vi "CAN_initialize_all.vi"() -> (3 "Array of Canopen Sessions":refnum<class "sbCANopenBaseClass.lvclass">[](array[class]), 6 "Array of Error out's":errorcluster[](array[cluster]))   [LabVIEW 2024]
uses:
  <vilib>/addons/Maxon Motor/EPOS2 CANopen/CANopen/sbCANopenBaseClass.lvclass
  <vilib>/addons/Maxon Motor/EPOS2 CANopen/EPOS2 Support Files/Typedefs/EPOS2 Config Data Input Current.ctl
  <vilib>/addons/Maxon Motor/EPOS2 CANopen/EPOS2 Support Files/Typedefs/EPOS2 Velocity Units.ctl
  <vilib>/addons/Maxon Motor/EPOS2 CANopen/EPOS2 Support Files/Typedefs/EPOS2 Control Word PVM.ctl
  <vilib>/addons/Maxon Motor/EPOS2 CANopen/EPOS2 Support Files/Polymorphic SubVIs/Config/EPOS2 Current Mode Configure.vi
  <vilib>/addons/Maxon Motor/EPOS2 CANopen/EPOS2 Support Files/Polymorphic SubVIs/Write PDO/EPOS2 Current Mode Write.vi
  <vilib>/addons/Maxon Motor/EPOS2 CANopen/EPOS2 Library.lvlib
  <vilib>/addons/Maxon Motor/EPOS2 CANopen/CANopen/CANopen IndCom Interface/sdCANopenIndCom.lvclass
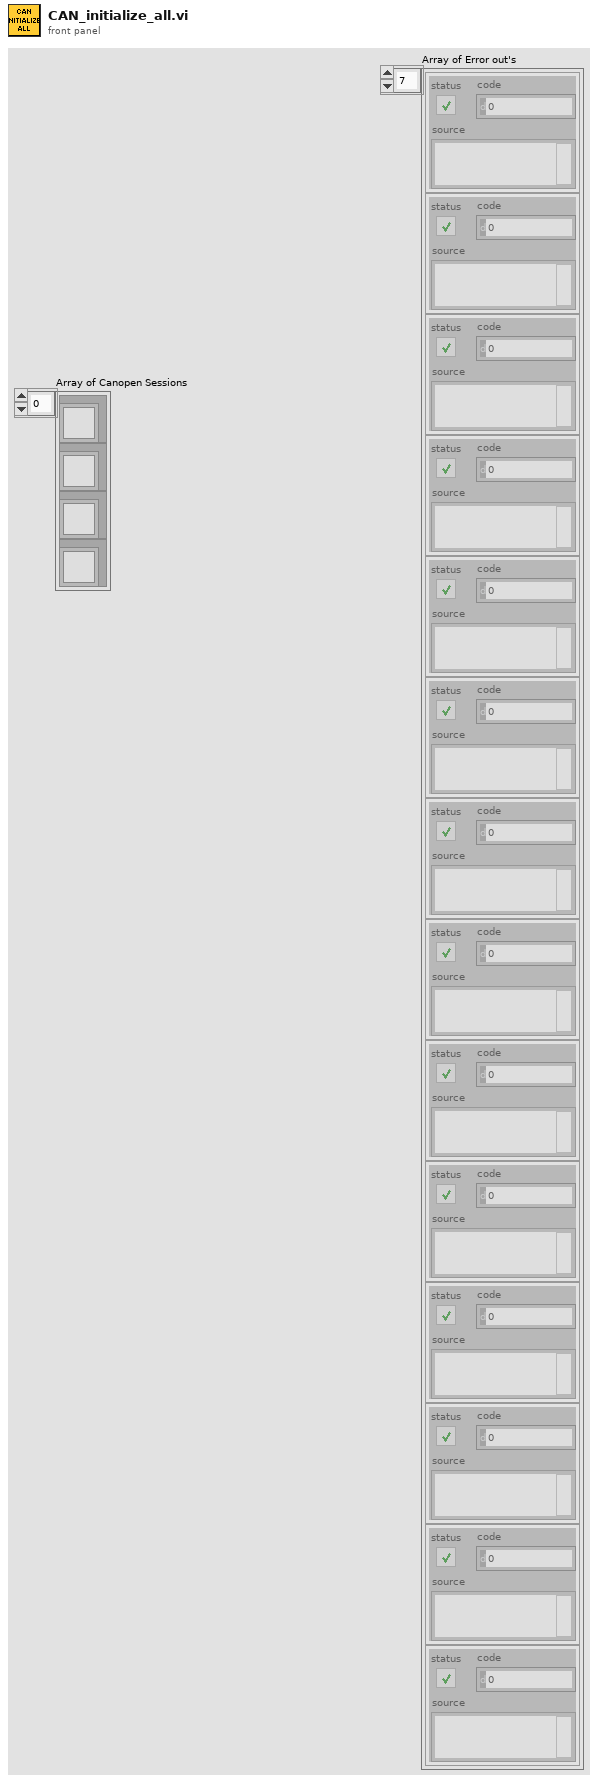
[diagram p1: front panel]
types:
  T1 = typedef "EPOS2 Library.lvlib/EPOS2 Control Word PVM.ctl" = cluster{"Switch On":bool, "Enable Voltage":bool, "Quick Stop":bool, "Enable Operation":bool, "Reserved 0":bool, "Reserved 1":bool, "Reserved 2":bool, "Fault Reset":bool, "Halt":bool}
  T2 = typedef "EPOS2 Library.lvlib/EPOS2 Config Data Input Current.ctl" = cluster{"Velocity Units":T3, "Max Velocity":i32}
  T3 = typedef "EPOS2 Library.lvlib/EPOS2 Velocity Units.ctl" = i8
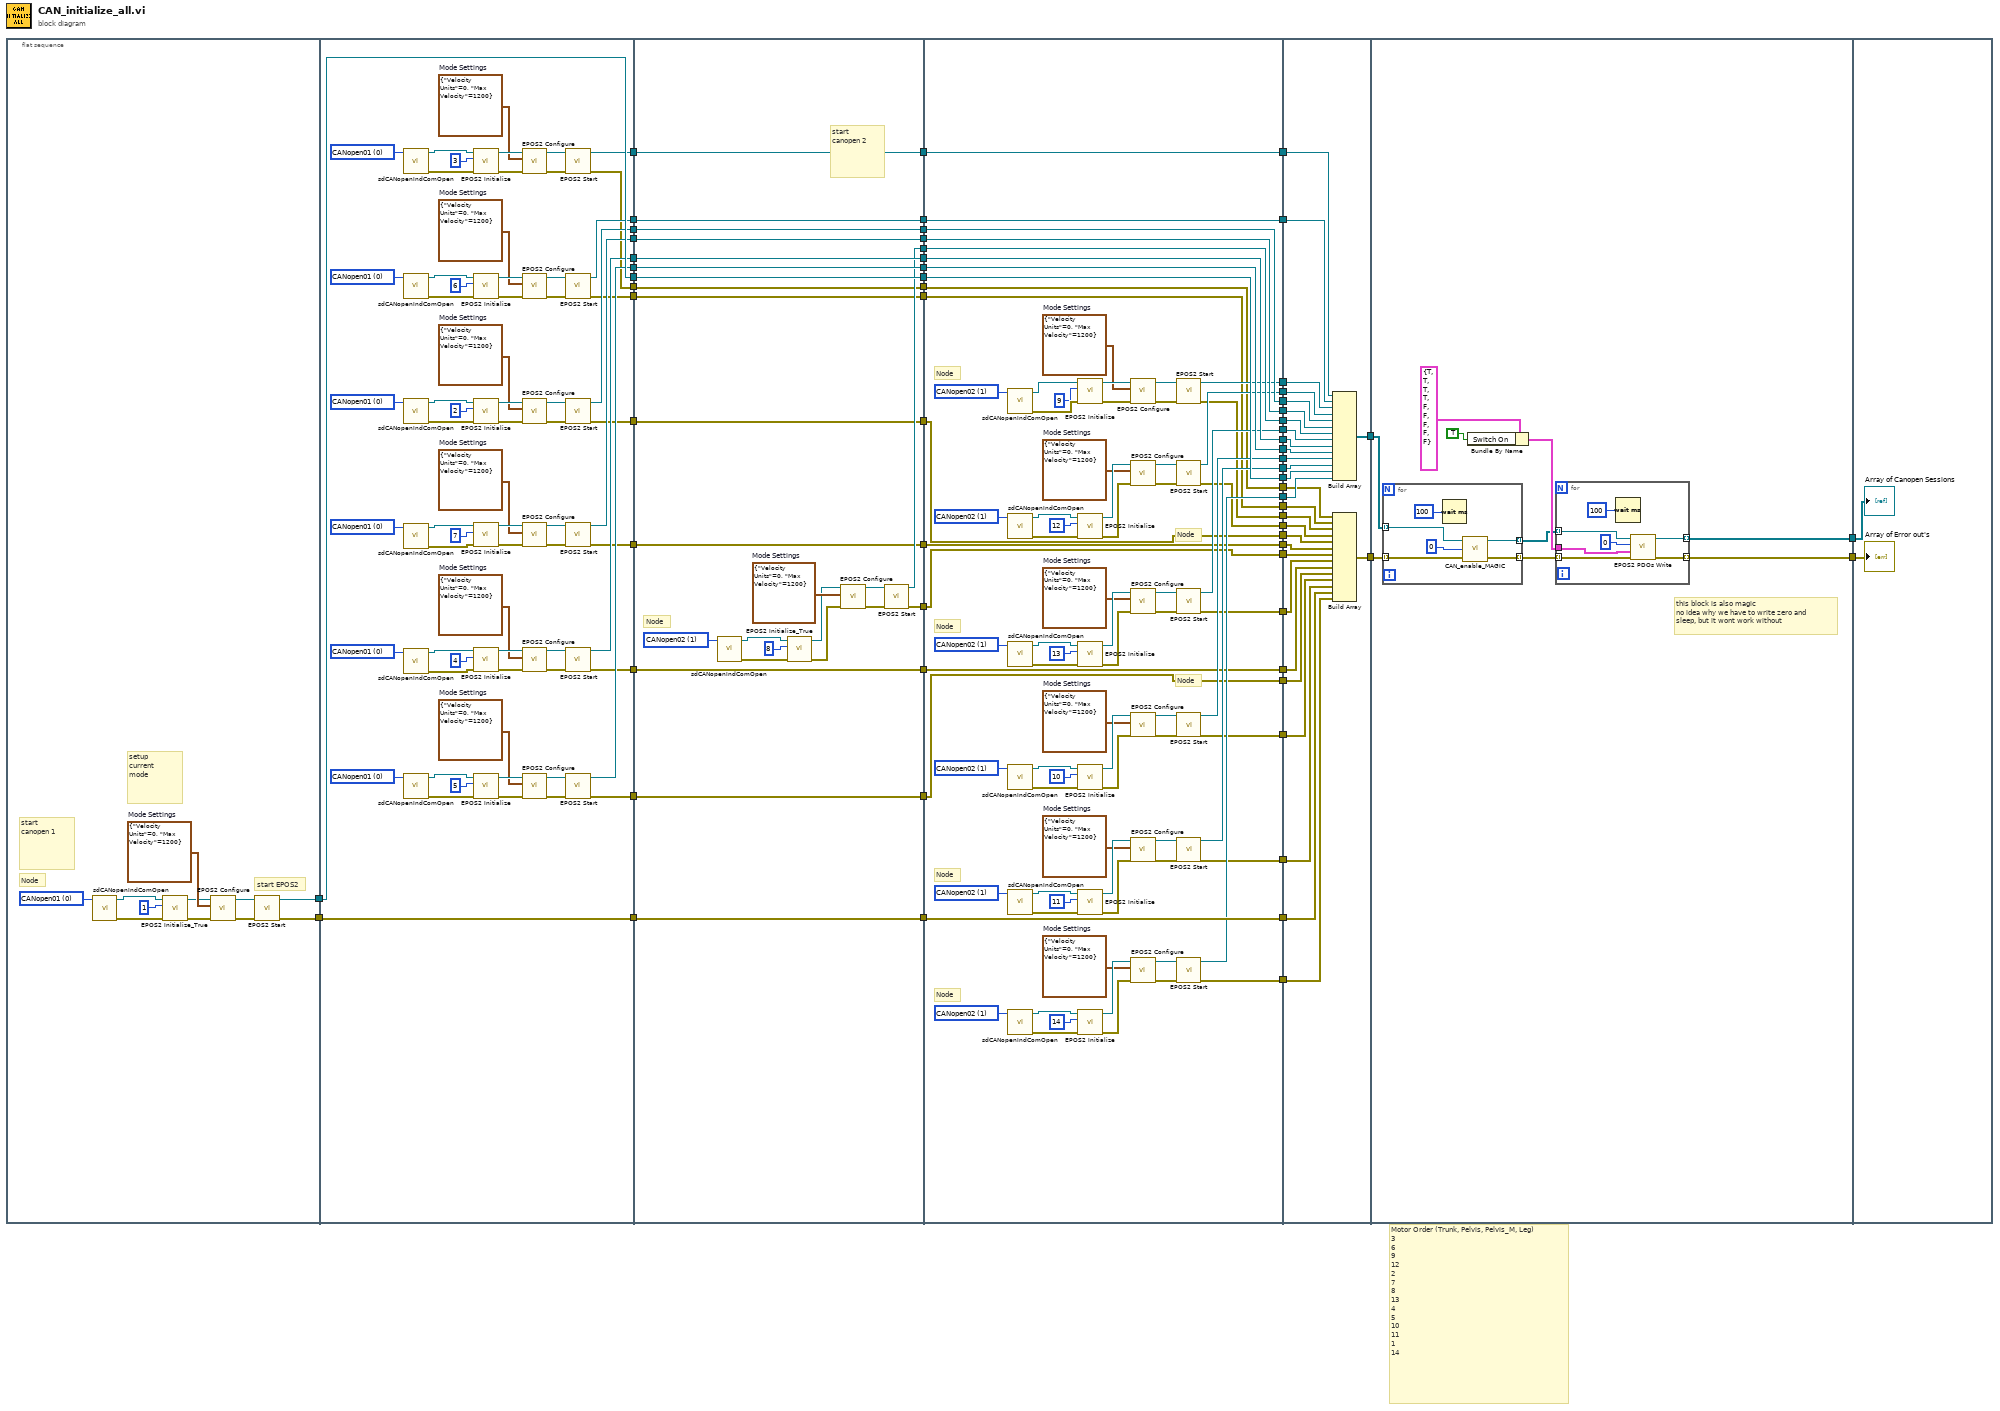
[diagram p0: block diagram]
diagram:
  # "Motor Order (Trunk, Pelvis, Pelvis_M, Leg)\n3\n6\n9\n12\n2\n7\n8\n13\n4\n5\n10\n11\n1\n14"
  n1 = flat-sequence {
    tunnel: [w66] -> w64
    tunnel: [w65] -> w60
    tunnel: w64 -> [w89]
    tunnel: [w89] -> w61
    tunnel: w60 -> [w88]
    tunnel: [w88] -> w57
    tunnel: [w87] -> w54
    tunnel: [w86] -> w53
    tunnel: [w85] -> w50
    tunnel: [w84] -> w47
    tunnel: [w83] -> w42
    tunnel: [w82] -> w39
    tunnel: [w81] -> w30
    tunnel: [w80] -> w25
    tunnel: [w79] -> w22
    tunnel: [w78] -> w19
    tunnel: [w77] -> w18
    tunnel: [w76] -> w14
    tunnel: [w159] -> w62
    tunnel: w61 -> [w159]
    tunnel: [w158] -> w58
    tunnel: w57 -> [w158]
    tunnel: [w157] -> w55
    tunnel: w54 -> [w157]
    tunnel: w53 -> [w156]
    tunnel: [w156] -> w51
    tunnel: w50 -> [w155]
    tunnel: [w155] -> w48
    tunnel: w47 -> [w154]
    tunnel: [w154] -> w45
    tunnel: [w153] -> w43
    tunnel: w42 -> [w153]
    tunnel: [w152] -> w40
    tunnel: w39 -> [w152]
    tunnel: [w151] -> w38
    tunnel: w30 -> [w150]
    tunnel: [w150] -> w28
    tunnel: [w149] -> w26
    tunnel: w25 -> [w149]
    tunnel: [w148] -> w23
    tunnel: w22 -> [w148]
    tunnel: [w147] -> w20
    tunnel: w19 -> [w147]
    tunnel: w18 -> [w146]
    tunnel: [w146] -> w16
    tunnel: [w145] -> w15
    tunnel: w14 -> [w145]
    tunnel: [w144] -> w12
    tunnel: [w196] -> w63
    tunnel: w62 -> [w196]
    tunnel: [w195] -> w59
    tunnel: w58 -> [w195]
    tunnel: [w194] -> w56
    tunnel: w55 -> [w194]
    tunnel: [w193] -> w52
    tunnel: w51 -> [w193]
    tunnel: [w192] -> w49
    tunnel: w48 -> [w192]
    tunnel: [w191] -> w46
    tunnel: w45 -> [w191]
    tunnel: [w190] -> w44
    tunnel: w43 -> [w190]
    tunnel: [w189] -> w41
    tunnel: w40 -> [w189]
    tunnel: w38 -> [w188]
    tunnel: [w188] -> w37
    tunnel: [w187] -> w36
    tunnel: [w186] -> w35
    tunnel: [w185] -> w34
    tunnel: [w184] -> w33
    tunnel: [w183] -> w32
    tunnel: [w182] -> w31
    tunnel: [w181] -> w29
    tunnel: w28 -> [w181]
    tunnel: [w180] -> w27
    tunnel: w26 -> [w180]
    tunnel: [w179] -> w24
    tunnel: w23 -> [w179]
    tunnel: [w178] -> w21
    tunnel: w20 -> [w178]
    tunnel: [w177] -> w17
    tunnel: w16 -> [w177]
    tunnel: w15 -> [w176]
    tunnel: [w176] -> w13
    tunnel: w12 -> [w175]
    tunnel: [w175] -> w11
    tunnel: [w174] -> w10
    tunnel: [w173] -> w9
    tunnel: [w172] -> w8
    tunnel: [w171] -> w7
    tunnel: [w170] -> w6
    tunnel: [w169] -> w5
    tunnel: w63 -> [w280]
    tunnel: w59 -> [w279]
    tunnel: w56 -> [w277]
    tunnel: w52 -> [w278]
    tunnel: w49 -> [w276]
    tunnel: w46 -> [w275]
    tunnel: w44 -> [w274]
    tunnel: w41 -> [w273]
    tunnel: w37 -> [w272]
    tunnel: w36 -> [w271]
    tunnel: w35 -> [w270]
    tunnel: w34 -> [w269]
    tunnel: w33 -> [w268]
    tunnel: w32 -> [w267]
    tunnel: w31 -> [w266]
    tunnel: w29 -> [w265]
    tunnel: w27 -> [w264]
    tunnel: w24 -> [w263]
    tunnel: w21 -> [w262]
    tunnel: w17 -> [w261]
    tunnel: w13 -> [w260]
    tunnel: w11 -> [w259]
    tunnel: w10 -> [w258]
    tunnel: w9 -> [w257]
    tunnel: w8 -> [w256]
    tunnel: w7 -> [w255]
    tunnel: w6 -> [w254]
    tunnel: w5 -> [w253]
    tunnel: [w252] -> w4
    tunnel: [w251] -> w3
    tunnel: w4 -> [w288]
    tunnel: w3 -> [w289]
    tunnel: [w282] -> w2
    tunnel: [w281] -> w1
    tunnel: w2 -> [w303]
    tunnel: w1 -> [w304]
    frame #0 {
      w74 = u32 0 items=["CANopen01", "CANopen02", "CANopen03", "CANopen04", "CANopen05", "CANopen06", "CANopen07", "CANopen08", "CANopen09", "CANopen10", "CANopen11", "CANopen12", "CANopen13", "CANopen14", "CANopen15", "CANopen16", "CANopen17", "CANopen18", "CANopen19", "CANopen20", "CANopen21", "CANopen22", "CANopen23", "CANopen24", "CANopen25", "CANopen26", "CANopen27", "CANopen28", "CANopen29", "CANopen30", "CANopen31", "CANopen32"] ("Interface Name")
      w75 = T2 {"Velocity Units"=0, "Max Velocity"=1200}  # Mode Settings
      # "start canopen 1"
      # "Node"
      # "start EPOS2"
      # "setup current mode"
      n2 = call <vilib>:"sdCANopenIndComOpen.vi"("Interface Name"=w74) -> ("error out"=w71:errorcluster, "SD CANopen Comm out"=w67:refnum<class "sbCANopenBaseClass.lvclass">)  [unwired: 9 in]
      n3 = call <vilib>:"EPOS2 Initialize_True.vi"("error in"=w71, "Node ID"=u8 1, "CAN Session In"=w67) -> ("error out"=w72:errorcluster, "CANopen Session Out"=w69:refnum<class "sbCANopenBaseClass.lvclass">)  [unwired: 7 in]
      n4 = call-poly <vilib>:"EPOS2 Configure.vi"("error in"=w72, "Mode Settings"=w75, "CANopen Session In"=w69) -> ("error out"=w70:errorcluster, "CANopen Session Out"=w68:refnum<class "sbCANopenBaseClass.lvclass">)  [unwired: 7 in]
      n5 = call <vilib>:"EPOS2 Start.vi"("error in"=w70, "CANopen Session In"=w68) -> ("error out"=w65:errorcluster, "CANopen Session Out"=w66:refnum<class "sbCANopenBaseClass.lvclass">)  [unwired: 8 in]
    }
    frame #1 {
      w93 = u32 0 items=["CANopen01", "CANopen02", "CANopen03", "CANopen04", "CANopen05", "CANopen06", "CANopen07", "CANopen08", "CANopen09", "CANopen10", "CANopen11", "CANopen12", "CANopen13", "CANopen14", "CANopen15", "CANopen16", "CANopen17", "CANopen18", "CANopen19", "CANopen20", "CANopen21", "CANopen22", "CANopen23", "CANopen24", "CANopen25", "CANopen26", "CANopen27", "CANopen28", "CANopen29", "CANopen30", "CANopen31", "CANopen32"] ("Interface Name")
      w94 = T2 {"Velocity Units"=0, "Max Velocity"=1200}  # Mode Settings
      w101 = u32 0 items=["CANopen01", "CANopen02", "CANopen03", "CANopen04", "CANopen05", "CANopen06", "CANopen07", "CANopen08", "CANopen09", "CANopen10", "CANopen11", "CANopen12", "CANopen13", "CANopen14", "CANopen15", "CANopen16", "CANopen17", "CANopen18", "CANopen19", "CANopen20", "CANopen21", "CANopen22", "CANopen23", "CANopen24", "CANopen25", "CANopen26", "CANopen27", "CANopen28", "CANopen29", "CANopen30", "CANopen31", "CANopen32"] ("Interface Name")
      w102 = T2 {"Velocity Units"=0, "Max Velocity"=1200}  # Mode Settings
      w113 = u32 0 items=["CANopen01", "CANopen02", "CANopen03", "CANopen04", "CANopen05", "CANopen06", "CANopen07", "CANopen08", "CANopen09", "CANopen10", "CANopen11", "CANopen12", "CANopen13", "CANopen14", "CANopen15", "CANopen16", "CANopen17", "CANopen18", "CANopen19", "CANopen20", "CANopen21", "CANopen22", "CANopen23", "CANopen24", "CANopen25", "CANopen26", "CANopen27", "CANopen28", "CANopen29", "CANopen30", "CANopen31", "CANopen32"] ("Interface Name")
      w114 = T2 {"Velocity Units"=0, "Max Velocity"=1200}  # Mode Settings
      w121 = u32 0 items=["CANopen01", "CANopen02", "CANopen03", "CANopen04", "CANopen05", "CANopen06", "CANopen07", "CANopen08", "CANopen09", "CANopen10", "CANopen11", "CANopen12", "CANopen13", "CANopen14", "CANopen15", "CANopen16", "CANopen17", "CANopen18", "CANopen19", "CANopen20", "CANopen21", "CANopen22", "CANopen23", "CANopen24", "CANopen25", "CANopen26", "CANopen27", "CANopen28", "CANopen29", "CANopen30", "CANopen31", "CANopen32"] ("Interface Name")
      w122 = T2 {"Velocity Units"=0, "Max Velocity"=1200}  # Mode Settings
      w129 = u32 0 items=["CANopen01", "CANopen02", "CANopen03", "CANopen04", "CANopen05", "CANopen06", "CANopen07", "CANopen08", "CANopen09", "CANopen10", "CANopen11", "CANopen12", "CANopen13", "CANopen14", "CANopen15", "CANopen16", "CANopen17", "CANopen18", "CANopen19", "CANopen20", "CANopen21", "CANopen22", "CANopen23", "CANopen24", "CANopen25", "CANopen26", "CANopen27", "CANopen28", "CANopen29", "CANopen30", "CANopen31", "CANopen32"] ("Interface Name")
      w130 = T2 {"Velocity Units"=0, "Max Velocity"=1200}  # Mode Settings
      w137 = u32 0 items=["CANopen01", "CANopen02", "CANopen03", "CANopen04", "CANopen05", "CANopen06", "CANopen07", "CANopen08", "CANopen09", "CANopen10", "CANopen11", "CANopen12", "CANopen13", "CANopen14", "CANopen15", "CANopen16", "CANopen17", "CANopen18", "CANopen19", "CANopen20", "CANopen21", "CANopen22", "CANopen23", "CANopen24", "CANopen25", "CANopen26", "CANopen27", "CANopen28", "CANopen29", "CANopen30", "CANopen31", "CANopen32"] ("Interface Name")
      w138 = T2 {"Velocity Units"=0, "Max Velocity"=1200}  # Mode Settings
      n6 = call <vilib>:"sdCANopenIndComOpen.vi"("Interface Name"=w129) -> ("error out"=w134:errorcluster, "SD CANopen Comm out"=w128:refnum<class "sbCANopenBaseClass.lvclass">)  [unwired: 9 in]
      n7 = call <vilib>:"sdCANopenIndComOpen.vi"("Interface Name"=w101) -> ("error out"=w106:errorcluster, "SD CANopen Comm out"=w100:refnum<class "sbCANopenBaseClass.lvclass">)  [unwired: 9 in]
      n8 = call <vilib>:"sdCANopenIndComOpen.vi"("Interface Name"=w137) -> ("error out"=w142:errorcluster, "SD CANopen Comm out"=w136:refnum<class "sbCANopenBaseClass.lvclass">)  [unwired: 9 in]
      n9 = call <vilib>:"sdCANopenIndComOpen.vi"("Interface Name"=w93) -> ("error out"=w98:errorcluster, "SD CANopen Comm out"=w92:refnum<class "sbCANopenBaseClass.lvclass">)  [unwired: 9 in]
      n10 = call <vilib>:"sdCANopenIndComOpen.vi"("Interface Name"=w121) -> ("error out"=w126:errorcluster, "SD CANopen Comm out"=w120:refnum<class "sbCANopenBaseClass.lvclass">)  [unwired: 9 in]
      n11 = call <vilib>:"sdCANopenIndComOpen.vi"("Interface Name"=w113) -> ("error out"=w118:errorcluster, "SD CANopen Comm out"=w112:refnum<class "sbCANopenBaseClass.lvclass">)  [unwired: 9 in]
      n12 = call <vilib>:"EPOS2 Initialize.vi"("error in"=w134, "Node ID"=u8 3, "CAN Session In"=w128) -> ("error out"=w135:errorcluster, "CANopen Session Out"=w132:refnum<class "sbCANopenBaseClass.lvclass">)  [unwired: 1 in, 6 out]
      n13 = call <vilib>:"EPOS2 Initialize.vi"("error in"=w106, "Node ID"=u8 6, "CAN Session In"=w100) -> ("error out"=w107:errorcluster, "CANopen Session Out"=w104:refnum<class "sbCANopenBaseClass.lvclass">)  [unwired: 1 in, 6 out]
      n14 = call <vilib>:"EPOS2 Initialize.vi"("error in"=w142, "Node ID"=u8 2, "CAN Session In"=w136) -> ("error out"=w143:errorcluster, "CANopen Session Out"=w140:refnum<class "sbCANopenBaseClass.lvclass">)  [unwired: 1 in, 6 out]
      n15 = call <vilib>:"EPOS2 Initialize.vi"("error in"=w98, "Node ID"=u8 7, "CAN Session In"=w92) -> ("error out"=w99:errorcluster, "CANopen Session Out"=w96:refnum<class "sbCANopenBaseClass.lvclass">)  [unwired: 1 in, 6 out]
      n16 = call <vilib>:"EPOS2 Initialize.vi"("error in"=w126, "Node ID"=u8 4, "CAN Session In"=w120) -> ("error out"=w127:errorcluster, "CANopen Session Out"=w124:refnum<class "sbCANopenBaseClass.lvclass">)  [unwired: 1 in, 6 out]
      n17 = call <vilib>:"EPOS2 Initialize.vi"("error in"=w118, "Node ID"=u8 5, "CAN Session In"=w112) -> ("error out"=w119:errorcluster, "CANopen Session Out"=w116:refnum<class "sbCANopenBaseClass.lvclass">)  [unwired: 1 in, 6 out]
      n18 = call-poly <vilib>:"EPOS2 Configure.vi"("error in"=w135, "Mode Settings"=w130, "CANopen Session In"=w132) -> ("error out"=w133:errorcluster, "CANopen Session Out"=w131:refnum<class "sbCANopenBaseClass.lvclass">)  [unwired: 7 in]
      n19 = call-poly <vilib>:"EPOS2 Configure.vi"("error in"=w107, "Mode Settings"=w102, "CANopen Session In"=w104) -> ("error out"=w105:errorcluster, "CANopen Session Out"=w103:refnum<class "sbCANopenBaseClass.lvclass">)  [unwired: 7 in]
      n20 = call-poly <vilib>:"EPOS2 Configure.vi"("error in"=w143, "Mode Settings"=w138, "CANopen Session In"=w140) -> ("error out"=w141:errorcluster, "CANopen Session Out"=w139:refnum<class "sbCANopenBaseClass.lvclass">)  [unwired: 7 in]
      n21 = call-poly <vilib>:"EPOS2 Configure.vi"("error in"=w99, "Mode Settings"=w94, "CANopen Session In"=w96) -> ("error out"=w97:errorcluster, "CANopen Session Out"=w95:refnum<class "sbCANopenBaseClass.lvclass">)  [unwired: 7 in]
      n22 = call-poly <vilib>:"EPOS2 Configure.vi"("error in"=w127, "Mode Settings"=w122, "CANopen Session In"=w124) -> ("error out"=w125:errorcluster, "CANopen Session Out"=w123:refnum<class "sbCANopenBaseClass.lvclass">)  [unwired: 7 in]
      n23 = call-poly <vilib>:"EPOS2 Configure.vi"("error in"=w119, "Mode Settings"=w114, "CANopen Session In"=w116) -> ("error out"=w117:errorcluster, "CANopen Session Out"=w115:refnum<class "sbCANopenBaseClass.lvclass">)  [unwired: 7 in]
      n24 = call <vilib>:"EPOS2 Start.vi"("error in"=w133, "CANopen Session In"=w131) -> ("error out"=w80:errorcluster, "CANopen Session Out"=w86:refnum<class "sbCANopenBaseClass.lvclass">)  [unwired: 8 in]
      n25 = call <vilib>:"EPOS2 Start.vi"("error in"=w105, "CANopen Session In"=w103) -> ("error out"=w77:errorcluster, "CANopen Session Out"=w83:refnum<class "sbCANopenBaseClass.lvclass">)  [unwired: 8 in]
      n26 = call <vilib>:"EPOS2 Start.vi"("error in"=w141, "CANopen Session In"=w139) -> ("error out"=w81:errorcluster, "CANopen Session Out"=w87:refnum<class "sbCANopenBaseClass.lvclass">)  [unwired: 8 in]
      n27 = call <vilib>:"EPOS2 Start.vi"("error in"=w97, "CANopen Session In"=w95) -> ("error out"=w76:errorcluster, "CANopen Session Out"=w82:refnum<class "sbCANopenBaseClass.lvclass">)  [unwired: 8 in]
      n28 = call <vilib>:"EPOS2 Start.vi"("error in"=w125, "CANopen Session In"=w123) -> ("error out"=w79:errorcluster, "CANopen Session Out"=w85:refnum<class "sbCANopenBaseClass.lvclass">)  [unwired: 8 in]
      n29 = call <vilib>:"EPOS2 Start.vi"("error in"=w117, "CANopen Session In"=w115) -> ("error out"=w78:errorcluster, "CANopen Session Out"=w84:refnum<class "sbCANopenBaseClass.lvclass">)  [unwired: 8 in]
    }
    frame #2 {
      w166 = u32 1 items=["CANopen01", "CANopen02", "CANopen03", "CANopen04", "CANopen05", "CANopen06", "CANopen07", "CANopen08", "CANopen09", "CANopen10", "CANopen11", "CANopen12", "CANopen13", "CANopen14", "CANopen15", "CANopen16", "CANopen17", "CANopen18", "CANopen19", "CANopen20", "CANopen21", "CANopen22", "CANopen23", "CANopen24", "CANopen25", "CANopen26", "CANopen27", "CANopen28", "CANopen29", "CANopen30", "CANopen31", "CANopen32"] ("Interface Name")
      w165 = T2 {"Velocity Units"=0, "Max Velocity"=1200}  # Mode Settings
      # "start canopen 2"
      # "Node"
      n30 = call <vilib>:"sdCANopenIndComOpen.vi"("Interface Name"=w166) -> ("error out"=w161:errorcluster, "SD CANopen Comm out"=w163:refnum<class "sbCANopenBaseClass.lvclass">)  [unwired: 9 in]
      n31 = call <vilib>:"EPOS2 Initialize_True.vi"("error in"=w161, "Node ID"=u8 8, "CAN Session In"=w163) -> ("error out"=w160:errorcluster, "CANopen Session Out"=w162:refnum<class "sbCANopenBaseClass.lvclass">)  [unwired: 7 in]
      n32 = call-poly <vilib>:"EPOS2 Configure.vi"("error in"=w160, "Mode Settings"=w165, "CANopen Session In"=w162) -> ("error out"=w167:errorcluster, "CANopen Session Out"=w168:refnum<class "sbCANopenBaseClass.lvclass">)  [unwired: 7 in]
      n33 = call <vilib>:"EPOS2 Start.vi"("error in"=w167, "CANopen Session In"=w168) -> ("error out"=w144:errorcluster, "CANopen Session Out"=w151:refnum<class "sbCANopenBaseClass.lvclass">)  [unwired: 8 in]
    }
    frame #3 {
      w205 = u32 1 items=["CANopen01", "CANopen02", "CANopen03", "CANopen04", "CANopen05", "CANopen06", "CANopen07", "CANopen08", "CANopen09", "CANopen10", "CANopen11", "CANopen12", "CANopen13", "CANopen14", "CANopen15", "CANopen16", "CANopen17", "CANopen18", "CANopen19", "CANopen20", "CANopen21", "CANopen22", "CANopen23", "CANopen24", "CANopen25", "CANopen26", "CANopen27", "CANopen28", "CANopen29", "CANopen30", "CANopen31", "CANopen32"] ("Interface Name")
      w204 = T2 {"Velocity Units"=0, "Max Velocity"=1200}  # Mode Settings
      w202 = u32 1 items=["CANopen01", "CANopen02", "CANopen03", "CANopen04", "CANopen05", "CANopen06", "CANopen07", "CANopen08", "CANopen09", "CANopen10", "CANopen11", "CANopen12", "CANopen13", "CANopen14", "CANopen15", "CANopen16", "CANopen17", "CANopen18", "CANopen19", "CANopen20", "CANopen21", "CANopen22", "CANopen23", "CANopen24", "CANopen25", "CANopen26", "CANopen27", "CANopen28", "CANopen29", "CANopen30", "CANopen31", "CANopen32"] ("Interface Name")
      w201 = T2 {"Velocity Units"=0, "Max Velocity"=1200}  # Mode Settings
      w199 = u32 1 items=["CANopen01", "CANopen02", "CANopen03", "CANopen04", "CANopen05", "CANopen06", "CANopen07", "CANopen08", "CANopen09", "CANopen10", "CANopen11", "CANopen12", "CANopen13", "CANopen14", "CANopen15", "CANopen16", "CANopen17", "CANopen18", "CANopen19", "CANopen20", "CANopen21", "CANopen22", "CANopen23", "CANopen24", "CANopen25", "CANopen26", "CANopen27", "CANopen28", "CANopen29", "CANopen30", "CANopen31", "CANopen32"] ("Interface Name")
      w198 = T2 {"Velocity Units"=0, "Max Velocity"=1200}  # Mode Settings
      w232 = u32 1 items=["CANopen01", "CANopen02", "CANopen03", "CANopen04", "CANopen05", "CANopen06", "CANopen07", "CANopen08", "CANopen09", "CANopen10", "CANopen11", "CANopen12", "CANopen13", "CANopen14", "CANopen15", "CANopen16", "CANopen17", "CANopen18", "CANopen19", "CANopen20", "CANopen21", "CANopen22", "CANopen23", "CANopen24", "CANopen25", "CANopen26", "CANopen27", "CANopen28", "CANopen29", "CANopen30", "CANopen31", "CANopen32"] ("Interface Name")
      w231 = T2 {"Velocity Units"=0, "Max Velocity"=1200}  # Mode Settings
      w229 = u32 1 items=["CANopen01", "CANopen02", "CANopen03", "CANopen04", "CANopen05", "CANopen06", "CANopen07", "CANopen08", "CANopen09", "CANopen10", "CANopen11", "CANopen12", "CANopen13", "CANopen14", "CANopen15", "CANopen16", "CANopen17", "CANopen18", "CANopen19", "CANopen20", "CANopen21", "CANopen22", "CANopen23", "CANopen24", "CANopen25", "CANopen26", "CANopen27", "CANopen28", "CANopen29", "CANopen30", "CANopen31", "CANopen32"] ("Interface Name")
      w228 = T2 {"Velocity Units"=0, "Max Velocity"=1200}  # Mode Settings
      w226 = u32 1 items=["CANopen01", "CANopen02", "CANopen03", "CANopen04", "CANopen05", "CANopen06", "CANopen07", "CANopen08", "CANopen09", "CANopen10", "CANopen11", "CANopen12", "CANopen13", "CANopen14", "CANopen15", "CANopen16", "CANopen17", "CANopen18", "CANopen19", "CANopen20", "CANopen21", "CANopen22", "CANopen23", "CANopen24", "CANopen25", "CANopen26", "CANopen27", "CANopen28", "CANopen29", "CANopen30", "CANopen31", "CANopen32"] ("Interface Name")
      w225 = T2 {"Velocity Units"=0, "Max Velocity"=1200}  # Mode Settings
      # "Node"
      # "Node"
      # "Node"
      # "Node"
      # "Node"
      # "Node"
      n34 = call <vilib>:"sdCANopenIndComOpen.vi"("Interface Name"=w226) -> ("error out"=w249:errorcluster, "SD CANopen Comm out"=w245:refnum<class "sbCANopenBaseClass.lvclass">)  [unwired: 9 in]
      n35 = call <vilib>:"sdCANopenIndComOpen.vi"("Interface Name"=w199) -> ("error out"=w222:errorcluster, "SD CANopen Comm out"=w218:refnum<class "sbCANopenBaseClass.lvclass">)  [unwired: 9 in]
      n36 = call <vilib>:"sdCANopenIndComOpen.vi"("Interface Name"=w202) -> ("error out"=w216:errorcluster, "SD CANopen Comm out"=w212:refnum<class "sbCANopenBaseClass.lvclass">)  [unwired: 9 in]
      n37 = call <vilib>:"sdCANopenIndComOpen.vi"("Interface Name"=w229) -> ("error out"=w243:errorcluster, "SD CANopen Comm out"=w239:refnum<class "sbCANopenBaseClass.lvclass">)  [unwired: 9 in]
      n38 = call <vilib>:"sdCANopenIndComOpen.vi"("Interface Name"=w232) -> ("error out"=w237:errorcluster, "SD CANopen Comm out"=w233:refnum<class "sbCANopenBaseClass.lvclass">)  [unwired: 9 in]
      n39 = call <vilib>:"sdCANopenIndComOpen.vi"("Interface Name"=w205) -> ("error out"=w210:errorcluster, "SD CANopen Comm out"=w206:refnum<class "sbCANopenBaseClass.lvclass">)  [unwired: 9 in]
      n40 = call <vilib>:"EPOS2 Initialize.vi"("error in"=w249, "Node ID"=u8 9, "CAN Session In"=w245) -> ("error out"=w250:errorcluster, "CANopen Session Out"=w247:refnum<class "sbCANopenBaseClass.lvclass">)  [unwired: 1 in, 6 out]
      n41 = call <vilib>:"EPOS2 Initialize.vi"("error in"=w222, "Node ID"=u8 12, "CAN Session In"=w218) -> ("error out"=w223:errorcluster, "CANopen Session Out"=w220:refnum<class "sbCANopenBaseClass.lvclass">)  [unwired: 1 in, 6 out]
      n42 = call <vilib>:"EPOS2 Initialize.vi"("error in"=w216, "Node ID"=u8 13, "CAN Session In"=w212) -> ("error out"=w217:errorcluster, "CANopen Session Out"=w214:refnum<class "sbCANopenBaseClass.lvclass">)  [unwired: 1 in, 6 out]
      n43 = call <vilib>:"EPOS2 Initialize.vi"("error in"=w243, "Node ID"=u8 10, "CAN Session In"=w239) -> ("error out"=w244:errorcluster, "CANopen Session Out"=w241:refnum<class "sbCANopenBaseClass.lvclass">)  [unwired: 1 in, 6 out]
      n44 = call <vilib>:"EPOS2 Initialize.vi"("error in"=w237, "Node ID"=u8 11, "CAN Session In"=w233) -> ("error out"=w238:errorcluster, "CANopen Session Out"=w235:refnum<class "sbCANopenBaseClass.lvclass">)  [unwired: 1 in, 6 out]
      n45 = call <vilib>:"EPOS2 Initialize.vi"("error in"=w210, "Node ID"=u8 14, "CAN Session In"=w206) -> ("error out"=w211:errorcluster, "CANopen Session Out"=w208:refnum<class "sbCANopenBaseClass.lvclass">)  [unwired: 1 in, 6 out]
      n46 = call-poly <vilib>:"EPOS2 Configure.vi"("error in"=w250, "Mode Settings"=w225, "CANopen Session In"=w247) -> ("error out"=w248:errorcluster, "CANopen Session Out"=w246:refnum<class "sbCANopenBaseClass.lvclass">)  [unwired: 7 in]
      n47 = call-poly <vilib>:"EPOS2 Configure.vi"("error in"=w223, "Mode Settings"=w198, "CANopen Session In"=w220) -> ("error out"=w221:errorcluster, "CANopen Session Out"=w219:refnum<class "sbCANopenBaseClass.lvclass">)  [unwired: 7 in]
      n48 = call-poly <vilib>:"EPOS2 Configure.vi"("error in"=w217, "Mode Settings"=w201, "CANopen Session In"=w214) -> ("error out"=w215:errorcluster, "CANopen Session Out"=w213:refnum<class "sbCANopenBaseClass.lvclass">)  [unwired: 7 in]
      n49 = call-poly <vilib>:"EPOS2 Configure.vi"("error in"=w244, "Mode Settings"=w228, "CANopen Session In"=w241) -> ("error out"=w242:errorcluster, "CANopen Session Out"=w240:refnum<class "sbCANopenBaseClass.lvclass">)  [unwired: 7 in]
      n50 = call-poly <vilib>:"EPOS2 Configure.vi"("error in"=w238, "Mode Settings"=w231, "CANopen Session In"=w235) -> ("error out"=w236:errorcluster, "CANopen Session Out"=w234:refnum<class "sbCANopenBaseClass.lvclass">)  [unwired: 7 in]
      n51 = call-poly <vilib>:"EPOS2 Configure.vi"("error in"=w211, "Mode Settings"=w204, "CANopen Session In"=w208) -> ("error out"=w209:errorcluster, "CANopen Session Out"=w207:refnum<class "sbCANopenBaseClass.lvclass">)  [unwired: 7 in]
      n52 = call <vilib>:"EPOS2 Start.vi"("error in"=w248, "CANopen Session In"=w246) -> ("error out"=w174:errorcluster, "CANopen Session Out"=w187:refnum<class "sbCANopenBaseClass.lvclass">)  [unwired: 8 in]
      n53 = call <vilib>:"EPOS2 Start.vi"("error in"=w221, "CANopen Session In"=w219) -> ("error out"=w171:errorcluster, "CANopen Session Out"=w184:refnum<class "sbCANopenBaseClass.lvclass">)  [unwired: 8 in]
      n54 = call <vilib>:"EPOS2 Start.vi"("error in"=w215, "CANopen Session In"=w213) -> ("error out"=w170:errorcluster, "CANopen Session Out"=w183:refnum<class "sbCANopenBaseClass.lvclass">)  [unwired: 8 in]
      n55 = call <vilib>:"EPOS2 Start.vi"("error in"=w242, "CANopen Session In"=w240) -> ("error out"=w173:errorcluster, "CANopen Session Out"=w186:refnum<class "sbCANopenBaseClass.lvclass">)  [unwired: 8 in]
      n56 = call <vilib>:"EPOS2 Start.vi"("error in"=w236, "CANopen Session In"=w234) -> ("error out"=w172:errorcluster, "CANopen Session Out"=w185:refnum<class "sbCANopenBaseClass.lvclass">)  [unwired: 8 in]
      n57 = call <vilib>:"EPOS2 Start.vi"("error in"=w209, "CANopen Session In"=w207) -> ("error out"=w169:errorcluster, "CANopen Session Out"=w182:refnum<class "sbCANopenBaseClass.lvclass">)  [unwired: 8 in]
    }
    frame #4 {
      n58 = Build Array(w278, w274, w271, w268, w277, w273, w272, w267, w276, w275, w270, w269, w280, w266) -> (w251:refnum<class "sbCANopenBaseClass.lvclass">[])
      n59 = Build Array(w264, w261, w258, w255, w265, w260, w259, w254, w263, w262, w257, w256, w279, w253) -> (w252:errorcluster[])
    }
    frame #5 {
      # "this block is also magic\nno idea why we have to write zero and\nsleep, but it wont work without"
      n60 = for {
        tunnel: [w300] -> w283 mode=indexing
        tunnel: [w299] -> w284 mode=indexing
        tunnel: w289 -> [w298] mode=indexing
        tunnel: w288 -> [w297] mode=indexing
        n61 = Wait (ms)(milliseconds to wait=u32 100) -> ()  [unwired: 1 out]
        n62 = call "CAN_enable_MAGIC.vi"("error in (no error)"=w297, "Current"=0, "sbCANopenBaseClass in"=w298) -> ("error out"=w299:errorcluster, "CANopen Session Out"=w300:refnum<class "sbCANopenBaseClass.lvclass">)  [unwired: 1 in]
      }
      n63 = Bundle By Name(cluster=T1 {"Switch On"=TRUE, "Enable Voltage"=TRUE, "Quick Stop"=TRUE, "Enable Operation"=TRUE, "Reserved 0"=FALSE, "Reserved 1"=FALSE, "Reserved 2"=FALSE, "Fault Reset"=FALSE, "Halt"=FALSE} ("Control Word"), "Switch On"=TRUE) -> (w285:T1)
      n64 = for {
        tunnel: w283 -> [w296] mode=indexing
        tunnel: w285 -> [w294]
        tunnel: w284 -> [w293] mode=indexing
        tunnel: [w290] -> w281 mode=indexing
        tunnel: [w291] -> w282 mode=indexing
        n65 = Wait (ms)(milliseconds to wait=u32 100) -> ()  [unwired: 1 out]
        n66 = call-poly <vilib>:"EPOS2 PDOs Write.vi"("error in"=w293, "Control Word"=w294, "Current"=0, "CANopen Session In"=w296) -> ("error out"=w290:errorcluster, "CANopen Session Out"=w291:refnum<class "sbCANopenBaseClass.lvclass">)  [unwired: 6 in]
      }
    }
    frame #6 {
      "Array of Error out's" <- w304
      "Array of Canopen Sessions" <- w303
    }
  }
